vi "Switch Tool.vi"(8 "error in (no error)":errorcluster, 11 "Main.lvlib:Main.lvclass":refnum<class "Main.lvclass">) -> (0 "error out":errorcluster, 3 "Main.lvlib:Main.lvclass 2":refnum<class "Main.lvclass">)   [LabVIEW 2018, in "Main.lvlib" / "Main.lvclass"]
uses:
  Main.lvclass
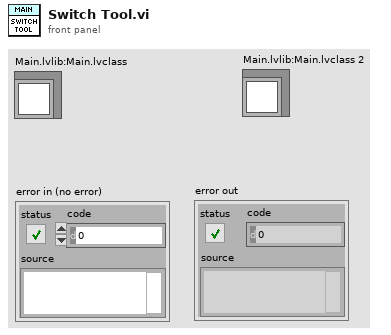
[diagram p1: front panel]
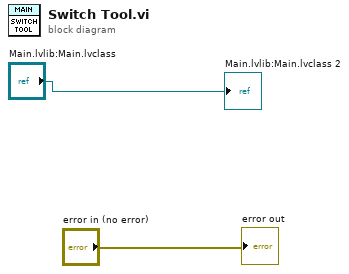
[diagram p0: block diagram]
diagram:
  "Main.lvlib:Main.lvclass 2" <- "Main.lvlib:Main.lvclass"
  "error out" <- "error in (no error)"
